vi "Input Multiplexer to FFT (4 inputs).vi"(7 "Reset?":bool, 8 "Input Data Valid Array":bool[](array[boolean])=[FALSE, FALSE, FALSE, FALSE], 11 "Input Data":i16[](array[numeric])=[0, 0, 0, 0]) -> (0 "Output Data Valid Array":bool[](array[boolean]), 3 "Interchanged Data":i16[](array[numeric]))   [LabVIEW 2011]
uses:
  <userlib>/FPGA Library/Code Development/Signal Processing/Input Multiplexer to FFT/4 Input MUX/Input Index(Type) 4 inputs.ctl
  <vilib>/rvi/FXPMathLib/basic elements/FxpDiscreteDelay/XNode/nifxpmath_DiscreteDelay.xnode
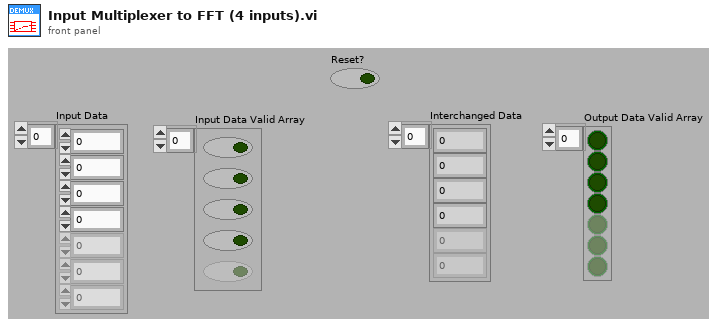
[diagram p1: front panel]
types:
  T1 = typedef "Input Index(Type) 4 inputs.ctl" = fxp<+,2,2>
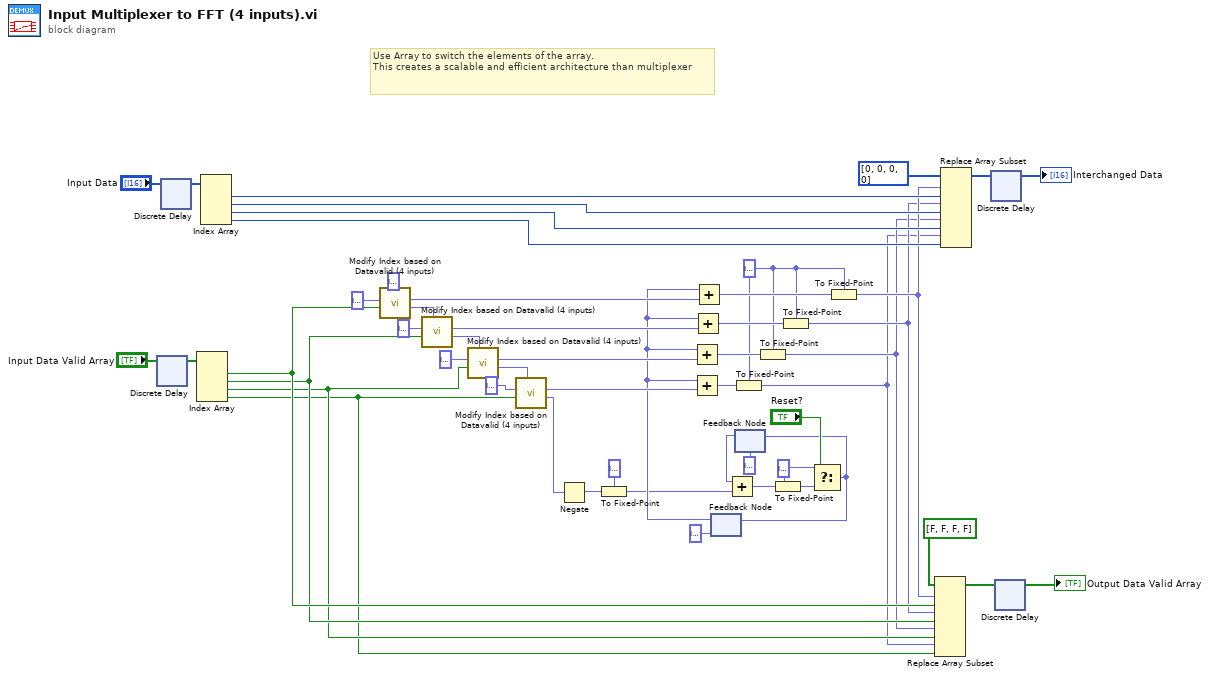
[diagram p0: block diagram]
diagram:
  w18 = T1 0.0
  w8 = T1 0.0 ("Actual Index")
  # "Use Array to switch the elements of the array. \nThis creates a scalable and efficient architecture than multiplexer"
  n1 = xnode "Discrete Delay"("D"="Input Data Valid Array") -> ("Q"=w4:bool[])
  n2 = xnode "Discrete Delay"("D"="Input Data") -> ("Q"=w3:i16[])
  n3 = Index Array(array=w4) -> (element #1=w44:bool, element #2=w43:bool, element #3=w42:bool, element #4=w41:bool)  [unwired: 4 in]
  n4 = Index Array(array=w3) -> (element #1=w31:i16, element #2=w30:i16, element #3=w29:i16, element #4=w28:i16)  [unwired: 4 in]
  n5 = call <userlib>:"Modify Index based on Datavalid (4 inputs).vi"("previous counter val"=T1 0.0, "cuurent index data valid?"=w44, "Actual Index"=T1 0.0) -> ("Next Counter Val"=w47:T1, "Modified Index"=w40:T1)  [unwired: 7 in]
  n6 = call <userlib>:"Modify Index based on Datavalid (4 inputs).vi"("previous counter val"=w47, "cuurent index data valid?"=w43, "Actual Index"=T1 1.0) -> ("Next Counter Val"=w46:T1, "Modified Index"=w38:T1)  [unwired: 7 in]
  n7 = call <userlib>:"Modify Index based on Datavalid (4 inputs).vi"("previous counter val"=w46, "cuurent index data valid?"=w42, "Actual Index"=T1 2.0) -> ("Next Counter Val"=w45:T1, "Modified Index"=w37:T1)  [unwired: 7 in]
  n8 = call <userlib>:"Modify Index based on Datavalid (4 inputs).vi"("previous counter val"=w45, "cuurent index data valid?"=w41, "Actual Index"=T1 3.0) -> ("Next Counter Val"=w20:T1, "Modified Index"=w36:T1)  [unwired: 7 in]
  n9 = Negate(x=w20) -> (-x=w12:fxp<+/-,3,3>)
  n10 = To Fixed-Point(fixed-point type=T1 0.0 ("Current Index Sum"), number=w12) -> (fixed-point=w11:T1)
  n11 = feedback #1(T1 0.0 ("Current Index Sum")) -> (w34:T1)
  n12 = Add(x=w34, y=w37) -> (x+y=w22:fxp<+,3,3>)
  n13 = Add(x=w34, y=w36) -> (x+y=w21:fxp<+,3,3>)
  n14 = Add(x=w34, y=w38) -> (x+y=w23:fxp<+,3,3>)
  n15 = Add(x=w34, y=w40) -> (x+y=w39:fxp<+,3,3>)
  n16 = To Fixed-Point(fixed-point type=w18, number=w21) -> (fixed-point=w13:T1)
  n17 = feedback #2(T1 0.0) -> (w33:T1)
  n18 = Add(x=w33, y=w11) -> (x+y=w19:fxp<+,3,3>)
  n19 = To Fixed-Point(fixed-point type=w18, number=w22) -> (fixed-point=w14:T1)
  n20 = To Fixed-Point(fixed-point type=w8, number=w19) -> (fixed-point=w9:T1)
  n21 = To Fixed-Point(fixed-point type=w18, number=w23) -> (fixed-point=w15:T1)
  n22 = Select(t=w8, s="Reset?", f=w9) -> (s? t:f=w6:T1)
  n23 = feedback-in #1(w6) -> ()
  n24 = feedback-in #2(w6) -> ()
  n25 = To Fixed-Point(fixed-point type=w18, number=w39) -> (fixed-point=w16:T1)
  n26 = Replace Array Subset(array=bool[] [FALSE, FALSE, FALSE, FALSE] ("appended array"), new element #1=w44, index #1=w16, new element #2=w43, index #2=w15, new element #3=w42, index #3=w14, new element #4=w41, index #4=w13) -> (w17:bool[])
  n27 = Replace Array Subset(array=i16[] [0, 0, 0, 0], new element #1=w31, index #1=w16, new element #2=w30, index #2=w15, new element #3=w29, index #3=w14, new element #4=w28, index #4=w13) -> (w25:i16[])
  n28 = xnode "Discrete Delay"("D"=w25) -> ("Q"=→"Interchanged Data":i16[])
  n29 = xnode "Discrete Delay"("D"=w17) -> ("Q"=→"Output Data Valid Array":bool[])
